vi "Documentos.vi"() -> ()   [LabVIEW 2019]
panel:
  in  "HOLD UP":bool
  in  "Testes":bool
  in  "Mapa Memória":bool
  in  "Tutorial Placa":bool
  in  "Merge":bool
  in  "Comunicacao":bool
  in  "stop":bool
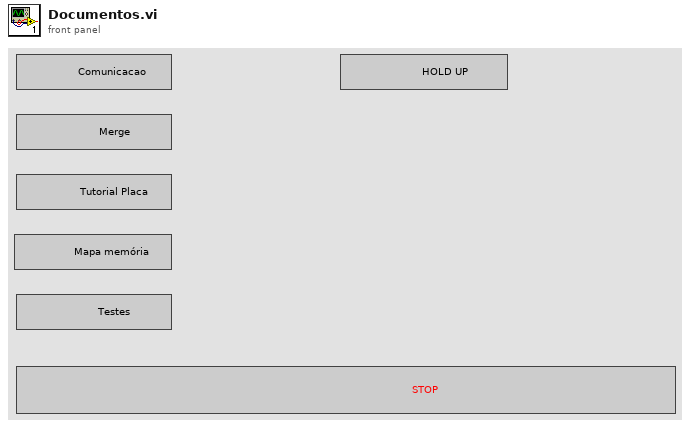
[diagram p1: front panel]
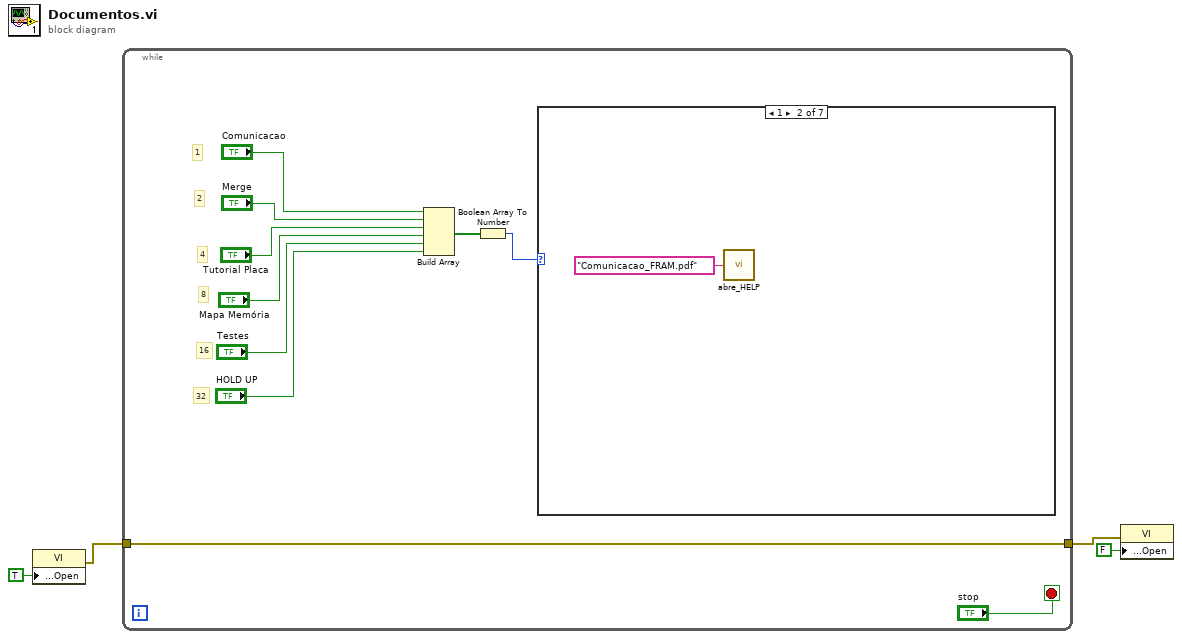
[diagram p0: block diagram]
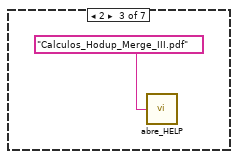
[diagram p3: hidden frame]
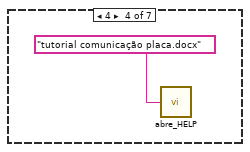
[diagram p4: hidden frame]
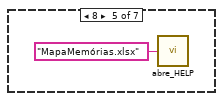
[diagram p5: hidden frame]
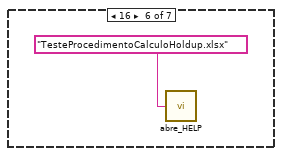
[diagram p6: hidden frame]
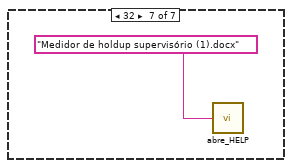
[diagram p7: hidden frame]
diagram:
  n1 = property class="VI"("Front Panel.Open"=TRUE ("Front Panel Window:Open")) -> (error out=w1:errorcluster)  [unwired: 2 in, 1 out]
  n2 = while {
    tunnel: [w13] -> w2
    tunnel: w1 -> [w13]
    stop <- "stop" stop-if-true
    # "32"
    # "16"
    # "8"
    # "4"
    # "2"
    # "1"
    n3 = Build Array("Comunicacao", "Merge", "Tutorial Placa", "Mapa Memória", "Testes", "HOLD UP") -> (w6:bool[])
    n4 = Boolean Array To Number(Boolean array=w6) -> (number=w5:u32)
    n5 = case shown="1" w5 {
      frame 0, Default {
      }
      frame 1 {
        n6 = call "abre_HELP.vi"("nome"="Comunicacao_FRAM.pdf") -> ()  [unwired: 1 out]
      }
      frame 2 {
        n7 = call "abre_HELP.vi"("nome"="Calculos_Hodup_Merge_III.pdf") -> ()  [unwired: 1 out]
      }
      frame 4 {
        n8 = call "abre_HELP.vi"("nome"="tutorial comunicação placa.docx") -> ()  [unwired: 1 out]
      }
      frame 8 {
        n9 = call "abre_HELP.vi"("nome"="MapaMemórias.xlsx") -> ()  [unwired: 1 out]
      }
      frame 16 {
        n10 = call "abre_HELP.vi"("nome"="TesteProcedimentoCalculoHoldup.xlsx") -> ()  [unwired: 1 out]
      }
      frame 32 {
        n11 = call "abre_HELP.vi"("nome"="Medidor de holdup supervisório (1).docx") -> ()  [unwired: 1 out]
      }
    }
  }
  n12 = property class="VI"(error in=w2, "Front Panel.Open"=FALSE ("Front Panel Window:Open")) -> ()  [unwired: 1 in, 2 out]
